vi "sub_SDR_mimo_rx.vi"(7 "System options":T1={"Samples per symbol"=6, "Roll-Off"=0.75, "Filter length (symbols)"=7, "Modulation Type"=enum."64-QAM", "Payload Symbols"=1472, "Symbols per Pilot"=6} {"Symbols per Pilot" min=6 max=16 step=2; "Payload Symbols" min=16 max=8192 step=16; "Filter length (symbols)" min=1 max=9 step=2; "Roll-Off" min=0.0 max=1.0 step=0.01; "Samples per symbol" min=2 max=32 step=2}, 10 "Radio Frame":cdb[][](array[numeric])) -> (0 "Constellation Data":cluster{dbl[], dbl[]}[](array[cluster]), 1 "Pilot SNR After equalization":dbl[](array[numeric]), 2 "SNR Before Equalizer":dbl[](array[numeric]), 3 "Received Packets in current frame":string[](array[string]), 4 "Received Data SNR":dbl[](array[numeric]))   [LabVIEW 2012]
panel:
  out "Last received packet num":i32
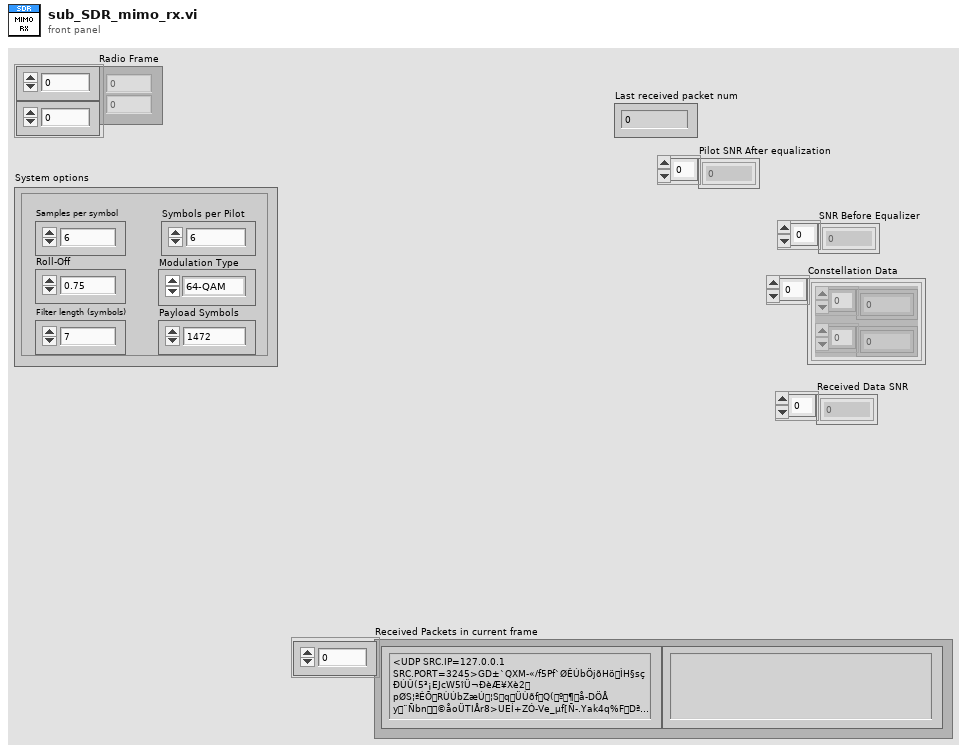
[diagram p1: front panel]
types:
  T1 = cluster{"Samples per symbol":i32, "Roll-Off":dbl, "Filter length (symbols)":i32, "Modulation Type":enum16{"BPSK", "4-QAM", "16-QAM", "64-QAM"}, "Payload Symbols":i32, "Symbols per Pilot":i32}
  T2 = cluster{"Samples per symbol":i32, "Roll-Off":dbl, "Filter length (symbols)":i32}
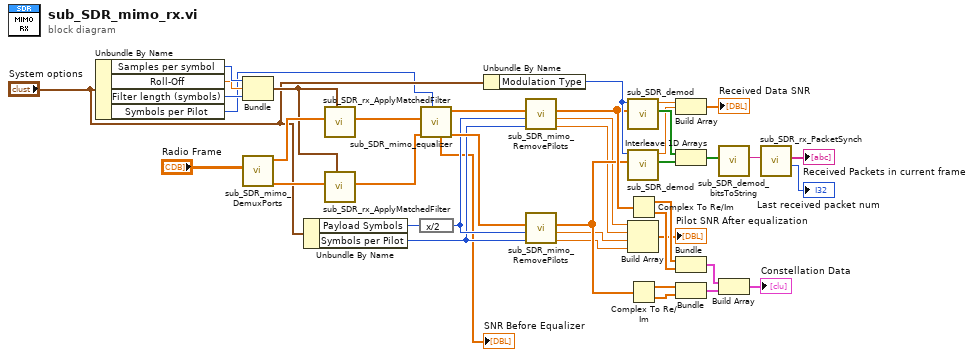
[diagram p0: block diagram]
diagram:
  n1 = Unbundle By Name("System options") -> ("Samples per symbol"=w22:i32, "Roll-Off"=w21:dbl, "Filter length (symbols)"=w20:i32, "Symbols per Pilot"=w15:i32)
  n2 = Bundle("Samples per symbol"=w22, "Roll-Off"=w21, "Filter length (symbols)"=w20) -> (w19:T2)  [unwired: 1 in]
  n3 = call "sub_SDR_mimo_DemuxPorts.vi"("Data in (2D)"="Radio Frame") -> ("Port 2"=w32:cdb[], "Port 1"=w31:cdb[])  [unwired: 9 in]
  n4 = Unbundle By Name("System options") -> ("Payload Symbols"=w18:i32, "Symbols per Pilot"=w14:i32)
  n5 = call "sub_SDR_rx_ApplyMatchedFilter.vi"("Filter Options"=w19, "Received stream"=w31) -> ("Received Symbols"=w29:cdb[])  [unwired: 9 in]
  n6 = call "sub_SDR_rx_ApplyMatchedFilter.vi"("Filter Options"=w19, "Received stream"=w32) -> ("Received Symbols"=w30:cdb[])  [unwired: 9 in]
  n7 = expression code="x/2"(w18) -> (w17:i32)
  n8 = call "sub_SDR_mimo_equalizer.vi"("Symbols per Pilot"=w15, "Input Symbols Port 2"=w30, "Input Symbols Port 1"=w29) -> ("Output symbols Port 2"=w34:cdb[], "Output symbols Port 1"=w33:cdb[], "SNR Before Equalizer"=→"SNR Before Equalizer":dbl[])  [unwired: 6 in]
  n9 = Unbundle By Name("System options") -> ("Modulation Type"=w35:enum16{"BPSK", "4-QAM", "16-QAM", "64-QAM"})
  n10 = call "sub_SDR_mimo_RemovePilots.vi"("Symbols per pilot"=w14, "Payload Symbols"=w17, "Array in"=w33) -> ("SNR 2 (dB)"=w4:dbl, "SNR 1 (dB)"=w5:dbl, "Array Out"=w13:cdb[])  [unwired: 6 in]
  n11 = call "sub_SDR_mimo_RemovePilots.vi"("Symbols per pilot"=w14, "Payload Symbols"=w17, "Array in"=w34) -> ("SNR 2 (dB)"=w2:dbl, "SNR 1 (dB)"=w3:dbl, "Array Out"=w12:cdb[])  [unwired: 6 in]
  n12 = call "sub_SDR_demod.vi"("Input Symbols"=w13, "Modulation Type"=w35) -> ("Output bits"=w37:bool[], "SNR [dB]"=w9:dbl)  [unwired: 8 in]
  n13 = call "sub_SDR_demod.vi"("Input Symbols"=w12, "Modulation Type"=w35) -> ("Output bits"=w36:bool[], "SNR [dB]"=w8:dbl)  [unwired: 8 in]
  n14 = Build Array(w5, w4, w3, w2) -> (→"Pilot SNR After equalization":dbl[])
  n15 = Complex To Re/Im(x + iy=w13) -> (x=w23:dbl[], y=w24:dbl[])
  n16 = Complex To Re/Im(x + iy=w12) -> (x=w26:dbl[], y=w27:dbl[])
  n17 = Build Array(w9, w8) -> (→"Received Data SNR":dbl[])
  n18 = Interleave 1D Arrays(w37, w36) -> (w38:bool[])
  n19 = Bundle(w23, w24) -> (w25:cluster{dbl[], dbl[]})  [unwired: 1 in]
  n20 = Bundle(w26, w27) -> (w28:cluster{dbl[], dbl[]})  [unwired: 1 in]
  n21 = call "sub_SDR_demod_bitsToString.vi"("Input bits"=w38) -> ("Output string"=w40:string)  [unwired: 10 in]
  n22 = Build Array(w25, w28) -> (→"Constellation Data":cluster{dbl[], dbl[]}[])
  n23 = call "sub_SDR_rx_PacketSynch.vi"("Input Stream"=w40) -> ("Last received packet num"=→"Last received packet num":i32, "Output Packets"=→"Received Packets in current frame":string[])  [unwired: 9 in]
